vi "WriteTausFile.vi"(7 "LVWSR":refnum<class "Web Request.lvclass">, 11 "Write_Data":u8) -> ()   [LabVIEW 2014]
uses:
  <vilib>/wsapi/Web Request.lvclass
  Controller/Messages/Stop Writing Taus MSG/Stop Writing Taus MSG.lvclass
  Controller/Messages/Start Tau Write MSG/Start Tau Write MSG.lvclass
  Controller/Controller.lvclass
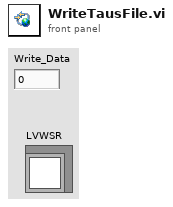
[diagram p1: front panel]
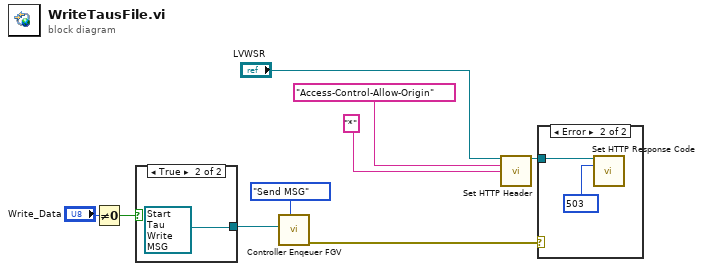
[diagram p0: block diagram]
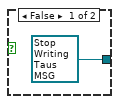
[diagram p2: hidden frame]
diagram:
  n1 = Not Equal To 0?(x="Write_Data") -> (x != 0?=w6:bool)
  n2 = case shown="True" w6 {
    tunnel: [refnum<class "Stop Writing Taus MSG.lvclass"> refnum ("Controller:Stop Writing Taus MSG.lvclass") refnum<class "Start Tau Write MSG.lvclass"> refnum ("Controller:Start Tau Write MSG.lvclass")] -> w5
    frame False {
    }
    frame True {
    }
  }
  n3 = call "Controller Enqeuer FGV.vi"("State"=enum16{"Store", "Send MSG"}."Send MSG", "MSG"=w5) -> ("error out"=w4:errorcluster)  [unwired: 9 in]
  n4 = call <vilib>:"Set HTTP Header.vi"("LabVIEW Web Service Request"="LVWSR", "header"="Access-Control-Allow-Origin", "header value"="*") -> ("LabVIEW Web Service Request out"=w7:refnum<class "Web Request.lvclass">)  [unwired: 11 in, 1 out]
  n5 = case shown="Error" w4 {
    tunnel: w7 -> [_ w13]
    frame No Error {
    }
    frame Error {
      w12 = 503 items=["100"=100, "101"=101, "200"=200, "201"=201, "202"=202, "203"=203, "204"=204, "205"=205, "206"=206, "300"=300, "301"=301, "302"=302, "303"=303, "304"=304, "305"=305, "306"=306, "307"=307, "400"=400, "401"=401, "402"=402, "403"=403, "404"=404, "405"=405, "406"=406, "407"=407, "408"=408, "409"=409, "410"=410, "411"=411, "412"=412, "413"=413, "414"=414, "415"=415, "416"=416, "417"=417, "500"=500, "501"=501, "502"=502, "503"=503, "504"=504, "505"=505] ("response code (200)")
      n6 = call <vilib>:"Set HTTP Response Code.vi"("LabVIEW Web Service Request"=w13, "response code (200)"=w12) -> ()  [unwired: 12 in, 2 out]
    }
  }
